vi "ReadTableBody.vi"(11 "tbodyString":string) -> (3 "tbodyData":string[][](array[string]))   [LabVIEW 2013]
uses:
  <vilib>/regexp/Match Regular Expression.xnode
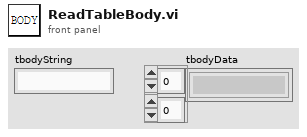
[diagram p1: front panel]
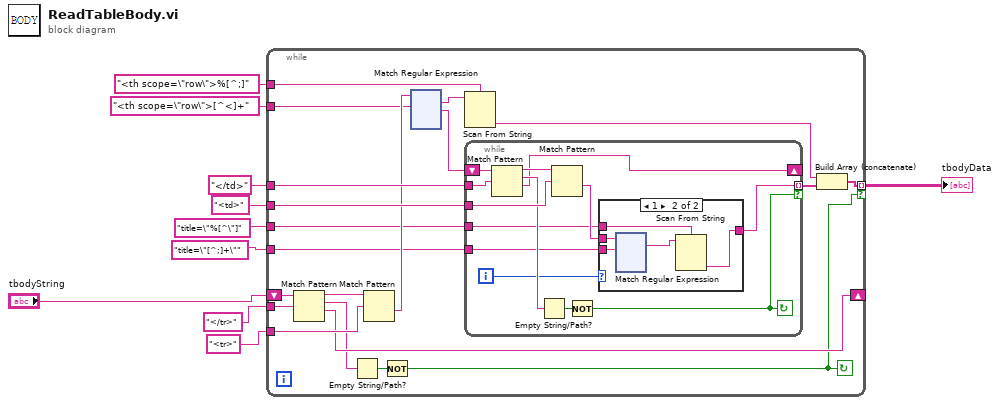
[diagram p0: block diagram]
diagram:
  n1 = while {
    shift-right: [w26] -> _
    shift-left: "tbodyString" -> [w30]
    tunnel: "</tr>" ("body") -> [w29]
    tunnel: "<tr>" ("body") -> [w27]
    tunnel: "</td>" ("body") -> [w24]
    tunnel: "<td>" ("body") -> [w23]
    tunnel: [w16] -> w10 mode=indexing if=w13
    tunnel: "<th scope=\"row\">[^<]+" ("body") -> [w20]
    tunnel: "<th scope=\"row\">%[^;]" ("body") -> [w18]
    tunnel: "title=\"%[^\"]" ("body") -> [w12]
    tunnel: "title=\"[^;]+\"" ("body") -> [w11]
    stop <- w13 continue-if-true
    n2 = Match Pattern(string=w30, regular expression=w29) -> (before substring=w28:string, match substring=w25:string, after substring=w26:string)  [unwired: 1 in, 1 out]
    n3 = Empty String/Path?(string/path=w25) -> (empty?=w14:bool)
    n4 = Match Pattern(string=w28, regular expression=w27) -> (after substring=w21:string)  [unwired: 1 in, 3 out]
    n5 = Not(x=w14) -> (.not. x?=w13:bool)
    n6 = xnode "Match Regular Expression"("input string"=w21, "regular expression"=w20) -> ("whole match"=w19:string, "after match"=w17:string)  [unwired: 4 in, 3 out]
    n7 = Scan From String(format string=w18, input string=w19) -> (output 1=w15:string)  [unwired: 3 in, 3 out]
    n8 = while {
      tunnel: w24 -> [w155]
      tunnel: w23 -> [w154]
      shift-right: [w152] -> _
      shift-left: w17 -> [w156]
      tunnel: [w147] -> w22 mode=indexing if=w150
      tunnel: w12 -> [w146]
      tunnel: w11 -> [w145]
      i -> [w149]
      stop <- w150 continue-if-true
      n9 = Match Pattern(string=w156, regular expression=w155) -> (before substring=w157:string, match substring=w153:string, after substring=w152:string)  [unwired: 1 in, 1 out]
      n10 = Empty String/Path?(string/path=w153) -> (empty?=w151:bool)
      n11 = Match Pattern(string=w157, regular expression=w154) -> (after substring=w148:string)  [unwired: 1 in, 3 out]
      n12 = Not(x=w151) -> (.not. x?=w150:bool)
      n13 = case shown="1" w149 {
        tunnel: [w158 w162] -> w147
        tunnel: w148 -> [w158 w161]
        tunnel: w146 -> [_ w163]
        tunnel: w145 -> [_ w159]
        frame Default {
        }
        frame 1 {
          n14 = xnode "Match Regular Expression"("input string"=w161, "regular expression"=w159) -> ("whole match"=w160:string)  [unwired: 4 in, 4 out]
          n15 = Scan From String(format string=w163, input string=w160) -> (output 1=w162:string)  [unwired: 3 in, 3 out]
        }
      }
    }
    n16 = Build Array (concatenate)(w15, w22) -> (w16:string[])
  }
  "tbodyData" <- w10
